vi "Periodic Tasks.vi"(8 "error in":errorcluster) -> ()   [LabVIEW 2019]
doc: "This VI runs in parallel to other tasks. It can contain as many user-defined periodic loops as you need. These can carry out PID or other sorts of timed response."
uses:
  <vilib>/Rock Robotics/WPI/Utilities/WPI_GetSetVariantRefNum.vi
  Robot Global Data.vi
  <vilib>/Rock Robotics/Network Tables/NT Write Number.vi
  <vilib>/Rock Robotics/WPI/RobotDrive/WPI_RobotDriveArcadeDrive_Standard(NoSaturation).vi
  <vilib>/Rock Robotics/Network Tables/NT Read Number.vi
  <vilib>/Rock Robotics/Network Tables/NT Read Boolean.vi
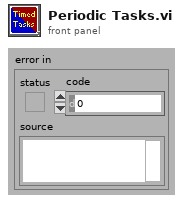
[diagram p1: front panel]
types:
  T1 = typedef "WPI_JoystickDevRef.ctl" = cluster{"Device":T2}
  T2 = typedef "WPI_JoystickDeviceEnum.ctl" = enum16{"USB 0", "USB 1", "USB 2", "USB 3", "USB 4", "USB 5"}
  T3 = typedef "WPI_RobotDriveDevRef.ctl" = cluster{"DevStatus":errorcluster, "Motors[]":T4[], "Square Inputs":bool, "Max Output":dbl}
  T4 = typedef "WPI_MotorControlDeviceRef.ctl" = cluster{"DeviceStatus":errorcluster, "Type":T5, "PWM":cluster{"PWM Channel":T6, "DeadBand":T7}, "CAN":cluster{"Device Number":u8, "SetOutput VI Ref":variant, "GetOutput VI Ref":variant, "Enable VI Ref":variant, "Disable VI Ref":variant, "Data":variant}, "Invert":bool, "DIO PWM":cluster{"PWM \"Enable\" Channel":T6, "DIOChannel":T8, "PWM Rate":dbl}}
  T5 = typedef "WPI_MotorControlType.ctl" = enum16{"PWM", "CAN", "DIO PWM"}
  T6 = typedef "FPGA_DIOPWMChannel.ctl" = enum8{"PWM 0", "PWM 1", "PWM 2", "PWM 3", "PWM 4", "PWM 5", "PWM 6", "PWM 7", "PWM 8", "PWM 9", "PWM MXP 0", "PWM MXP 1", "PWM MXP 2", "PWM MXP 3", "PWM MXP 4", "PWM MXP 5", "PWM MXP 6", "PWM MXP 7", "PWM MXP 8", "PWM MXP 9", "Invalid"}
  T7 = typedef "WPI_PWMDeadband.ctl" = cluster{"Name":string, "maxPositivePwm":i32, "minPositivePwm":i32, "centerPwm":i32, "maxNegativePwm":i32, "minNegativePwm":i32, "angularRange":u16}
  T8 = typedef "FPGA_DIOChannel.ctl" = enum8{"DIO 0", "DIO 1", "DIO 2", "DIO 3", "DIO 4", "DIO 5", "DIO 6", "DIO 7", "DIO 8", "DIO 9", "DIO MXP 0", "DIO MXP 1", "DIO MXP 2", "DIO MXP 3", "DIO MXP 4", "DIO MXP 5", "DIO MXP 6", "DIO MXP 7", "DIO MXP 8", "DIO MXP 9", "DIO MXP 10", "DIO MXP 11", "DIO MXP 12", "DIO MXP 13", "DIO MXP 14", "DIO MXP 15", "SPI Port CS1", "SPI Port CS2", "SPI Port CS3", "SPI Port MISO", "SPI Port MOSI", "Invalid"}
  T9 = cluster{"JoystickDevRef":T1, "RobotDriveDevRef":T3}
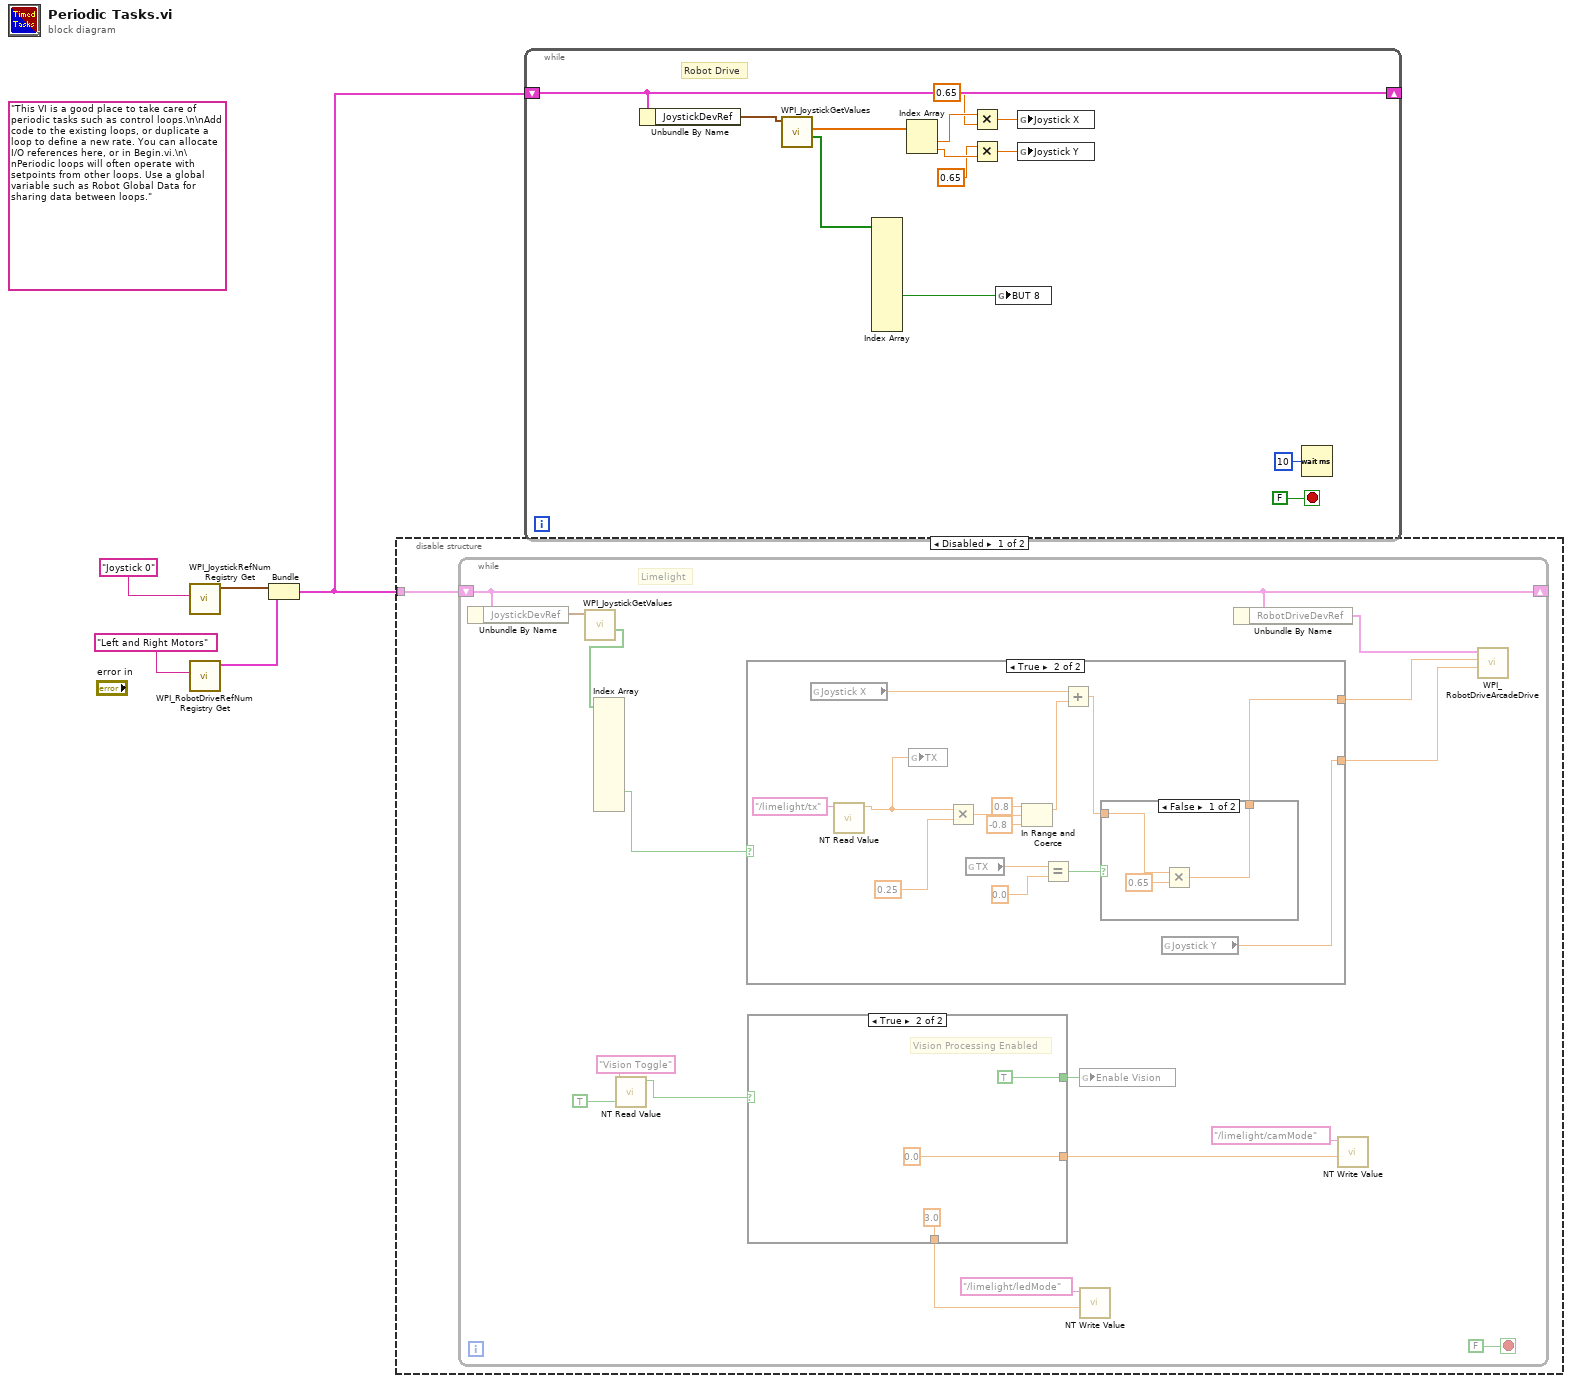
[diagram p0: block diagram]
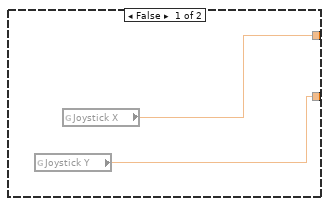
[diagram p2: hidden frame]
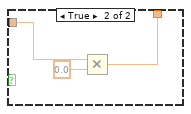
[diagram p3: hidden frame]
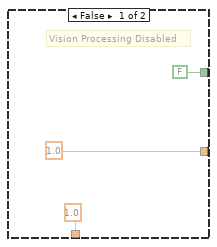
[diagram p4: hidden frame]
diagram:
  (unwired) "This VI is a good place to take care of periodic tasks such as control loops.\n\nAdd code to the existing loops, or duplicate a loop to define a new rate. You can allocate I/O references here, or in Begin.vi.\n\nPeriodic loops will often operate with setpoints from other loops. Use a global variable such as Robot Global Data for sharing data between loops."
  n1 = call <vilib>:"WPI_JoystickRefNum Registry Get.vi"("refnum name"="Joystick 0") -> ("JoystickDevRef"=w3:T1)  [unwired: 1 in, 9 out]
  n2 = call <vilib>:"WPI_RobotDriveRefNum Registry Get.vi"("refnum name"="Left and Right Motors") -> ("RobotDriveDevRef"=w2:T3)  [unwired: 1 in, 9 out]
  n3 = Bundle("JoystickDevRef"=w3, "RobotDriveDevRef"=w2) -> (w1:T9)  [unwired: 1 out]
  n4 = disable-structure shown="Disabled" {
    disable-tunnel: w1 -> [w6 _]
    frame Disabled {
      n5 = while {
        shift-right: [w18] -> _
        shift-left: w6 -> [w18]
        stop <- FALSE stop-if-true
        # "Limelight"
        n6 = Unbundle By Name(w18) -> ("JoystickDevRef"=w17:T1)
        n7 = call <vilib>:"WPI_JoystickGetValues.vi"("JoystickDevRef"=w17) -> ("Buttons"=w16:bool[])  [unwired: 6 in, 4 out]
        n8 = Index Array(array=w16) -> (element #10=w10:bool)  [unwired: 12 in, 11 out]
        n9 = call-poly <vilib>:"NT Read Value.vi"("Default Value"=TRUE, "Name"="Vision Toggle") -> ("Boolean"=w9:bool)  [unwired: 8 in, 1 out]
        n10 = case shown="True" w10 {
          tunnel: [w24 w29] -> w19
          tunnel: [w23 w25] -> w7
          frame False {
            n11 = global read "Robot Global Data.vi" "Joystick Y"() -> (w23:dbl)
            n12 = global read "Robot Global Data.vi" "Joystick X"() -> (w24:dbl)
          }
          frame True {
            n13 = global read "Robot Global Data.vi" "Joystick X"() -> (w37:dbl)
            n14 = call-poly <vilib>:"NT Read Value.vi"("Name"="/limelight/tx") -> ("Numeric"=w31:dbl)  [unwired: 9 in, 1 out]
            n15 = global write "Robot Global Data.vi" "TX"(w31) -> ()
            n16 = Multiply(x=w31, y=0.25) -> (x*y=w35:dbl)
            n17 = global read "Robot Global Data.vi" "TX"() -> (w27:dbl)
            n18 = In Range and Coerce(upper limit=0.8, x=w35, lower limit=-0.8) -> (coerced(x)=w36:dbl)  [unwired: 1 out]
            n19 = Equal?(x=w27, y=0.0) -> (x = y?=w28:bool)
            n20 = Add(x=w37, y=w36) -> (x+y=w30:dbl)
            n21 = case shown="False" w28 {
              tunnel: w30 -> [w40 w44]
              tunnel: [w41 w42] -> w29
              frame False {
                n22 = Multiply(x=w40, y=0.65) -> (x*y=w41:dbl)
              }
              frame True {
                n23 = Multiply(x=w44, y=0.0) -> (x*y=w42:dbl)
              }
            }
            n24 = global read "Robot Global Data.vi" "Joystick Y"() -> (w25:dbl)
          }
        }
        n25 = case shown="True" w9 {
          tunnel: [FALSE ("Enable Vision") TRUE ("Enable Vision")] -> w21
          tunnel: [1.0 ("Numeric") 0.0 ("Numeric")] -> w14
          tunnel: [1.0 ("Numeric") 3.0 ("Numeric")] -> w11
          frame False {
            # "Vision Processing Disabled"
          }
          frame True {
            # "Vision Processing Enabled"
          }
        }
        n26 = global write "Robot Global Data.vi" "Enable Vision"(w21) -> ()
        n27 = call-poly <vilib>:"NT Write Value.vi"("Numeric"=w11, "Name"="/limelight/ledMode") -> ()  [unwired: 9 in, 1 out]
        n28 = Unbundle By Name(w18) -> ("RobotDriveDevRef"=w20:T3)
        n29 = call-poly <vilib>:"NT Write Value.vi"("Numeric"=w14, "Name"="/limelight/camMode") -> ()  [unwired: 9 in, 1 out]
        n30 = call-poly <vilib>:"WPI_RobotDriveArcadeDrive.vi"("Y axis value"=w7, "X axis value"=w19, "RobotDriveDevRef"=w20) -> ()  [unwired: 6 in, 3 out]
      }
    }
    frame Enabled {
    }
  }
  n31 = while {
    shift-right: [w62] -> _
    shift-left: w1 -> [w62]
    stop <- FALSE stop-if-true
    # "Robot Drive"
    n32 = Unbundle By Name(w62) -> ("JoystickDevRef"=w60:T1)
    n33 = call <vilib>:"WPI_JoystickGetValues.vi"("JoystickDevRef"=w60) -> ("Buttons"=w52:bool[], "Axes"=w59:dbl[])  [unwired: 6 in, 3 out]
    n34 = Index Array(array=w52) -> (element #8=w51:bool)  [unwired: 12 in, 11 out]
    n35 = Index Array(array=w59) -> (element #1=w58:dbl, element #2=w56:dbl)  [unwired: 2 in]
    n36 = Multiply(x=w58, y=0.65) -> (x*y=w54:dbl)
    n37 = Multiply(x=0.65, y=w56) -> (x*y=w53:dbl)
    n38 = global write "Robot Global Data.vi" "BUT 8"(w51) -> ()
    n39 = global write "Robot Global Data.vi" "Joystick X"(w54) -> ()
    n40 = global write "Robot Global Data.vi" "Joystick Y"(w53) -> ()
    n41 = Wait (ms)(milliseconds to wait=u32 10) -> ()  [unwired: 1 out]
  }
